vi "Signal_Generator.vi"() -> ()   [LabVIEW 2019]
panel:
  in  "TriangleCounter":u32
  in  "Fire":bool
  in  "Duty (percentage)":dbl
  in  "Period (ms)":u32
  in  "Channel":string(combo)
  in  "Signal Type":string(combo)
  out "esdaqErrorOut":errorcluster
  in  "esdaqPortInp":refnum<visa-resource-name>
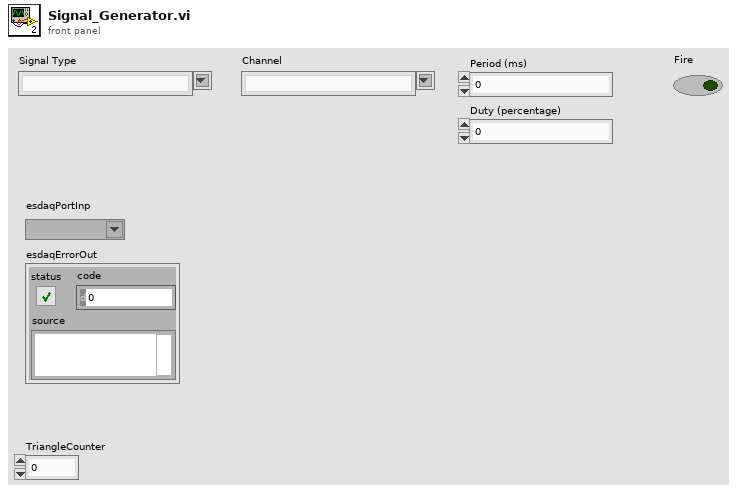
[diagram p1: front panel]
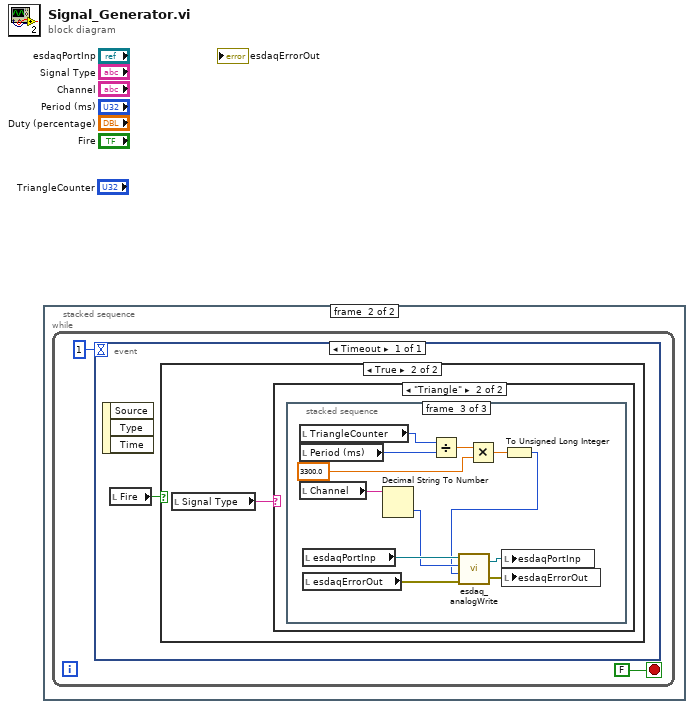
[diagram p0: block diagram]
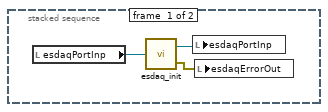
[diagram p2: hidden frame]
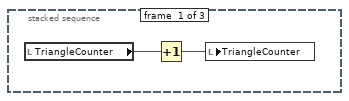
[diagram p5: hidden frame]
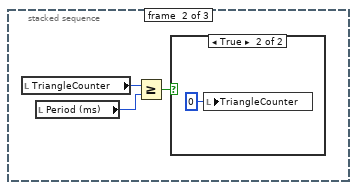
[diagram p6: hidden frame]
diagram:
  n1 = stacked-sequence {
    frame #0 {
      n2 = local read "esdaqPortInp"() -> (w2:refnum<visa-resource-name>)
      n3 = call "esdaq_init.vi"("esdaqPortInp"=w2) -> ("esdaqPortOut"=w3:refnum<visa-resource-name>, "esdaqErrorOut"=w1:errorcluster)
      n4 = local write "esdaqPortInp"(w3) -> ()
      n5 = local write "esdaqErrorOut"(w1) -> ()
    }
    frame #1 {
      n6 = while {
        stop <- FALSE stop-if-true
        n7 = event shown="[0] Timeout" {
          selector: _ -> [_]
          dyn-events: _ -> [_]
          timeout: 1 -> [_]
          event Timeout {
            n8 = event-data() -> ()  [unwired: 1 in, 3 out]
            n9 = local read "Fire"() -> (w6:bool)
            n10 = case shown="True" w6 {
              frame False {
              }
              frame True {
                n11 = local read "Signal Type"() -> (w7:string)
                n12 = case shown="\"Triangle\"" w7 {
                  frame "False", Default {
                  }
                  frame "Triangle" {
                    n13 = stacked-sequence {
                      frame #0 {
                        n14 = local read "TriangleCounter"() -> (w9:u32)
                        n15 = Increment(x=w9) -> (x+1=w8:u32)
                        n16 = local write "TriangleCounter"(w8) -> ()
                      }
                      frame #1 {
                        n17 = local read "TriangleCounter"() -> (w11:u32)
                        n18 = local read "Period (ms)"() -> (w12:u32)
                        n19 = Greater Or Equal?(x=w11, y=w12) -> (x >= y?=w10:bool)
                        n20 = case shown="True" w10 {
                          frame False {
                          }
                          frame True {
                            n21 = local write "TriangleCounter"(u32 0 ("TriangleCounter")) -> ()
                          }
                        }
                      }
                      frame #2 {
                        n22 = local read "TriangleCounter"() -> (w23:u32)
                        n23 = local read "Period (ms)"() -> (w22:u32)
                        n24 = local read "Channel"() -> (w20:string)
                        n25 = local read "esdaqPortInp"() -> (w19:refnum<visa-resource-name>)
                        n26 = local read "esdaqErrorOut"() -> (w18:errorcluster)
                        n27 = Decimal String To Number(string=w20) -> (number=w15:i32)  [unwired: 2 in, 1 out]
                        n28 = Divide(x=w23, y=w22) -> (x/y=w25:dbl)
                        n29 = Multiply(x=w25, y=3300.0) -> (x*y=w21:dbl)
                        n30 = To Unsigned Long Integer(number=w21) -> (unsigned 32bit integer=w14:u32)
                        n31 = call "esdaq_analogWrite.vi"("esdaqErrorInp"=w18, "Value"=w14, "Channel"=w15, "esdaqPortInp"=w19) -> ("esdaqErrorOut"=w17:errorcluster, "esdaqPortOut"=w16:refnum<visa-resource-name>)
                        n32 = local write "esdaqPortInp"(w16) -> ()
                        n33 = local write "esdaqErrorOut"(w17) -> ()
                      }
                    }
                  }
                }
              }
            }
          }
        }
      }
    }
  }
